vi "Add_Update_Values.vi"(0 "Filename":path, 1 "Value  Constant?":bool, 2 "Edit Raw data files?":bool, 3 "Filetype":string, 5 "New Chs In":string[](array[string])=[""], 7 "Edit Raw Data Header Info":bool, 9 "New Values In":string[][](array[string]), 11 "Selected Rows":i32[](array[numeric]), 12 "Edit all Rows?":bool, 13 "Raw DF in Orig Pos?":bool, 14 "Job Directory":path=path "/G4_2_HD/Users/paulhayden/Documents/Projects/Hong Roughness/XW data/XW_Corr.tpt") -> ()   [LabVIEW 2015]
panel:
  in  "Warn If files not found?":bool=TRUE
  out "Checking Raw data files":i32
  in  "stop":bool
  out "Currently editing":string
  out "Folder Containing Raw data Files":path
  out "size(s)":i32
  out "Files Processed":i32(slide) scale=0.0..522.0
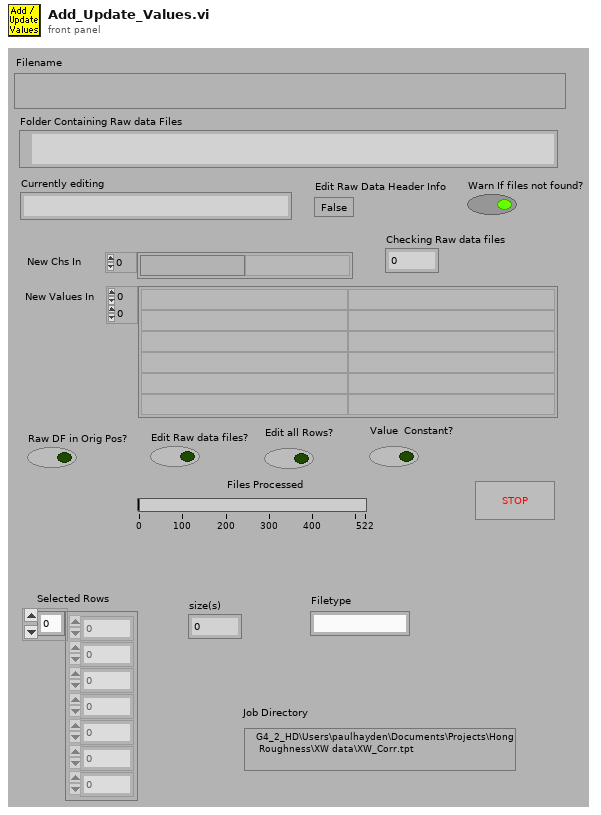
[diagram p1: front panel]
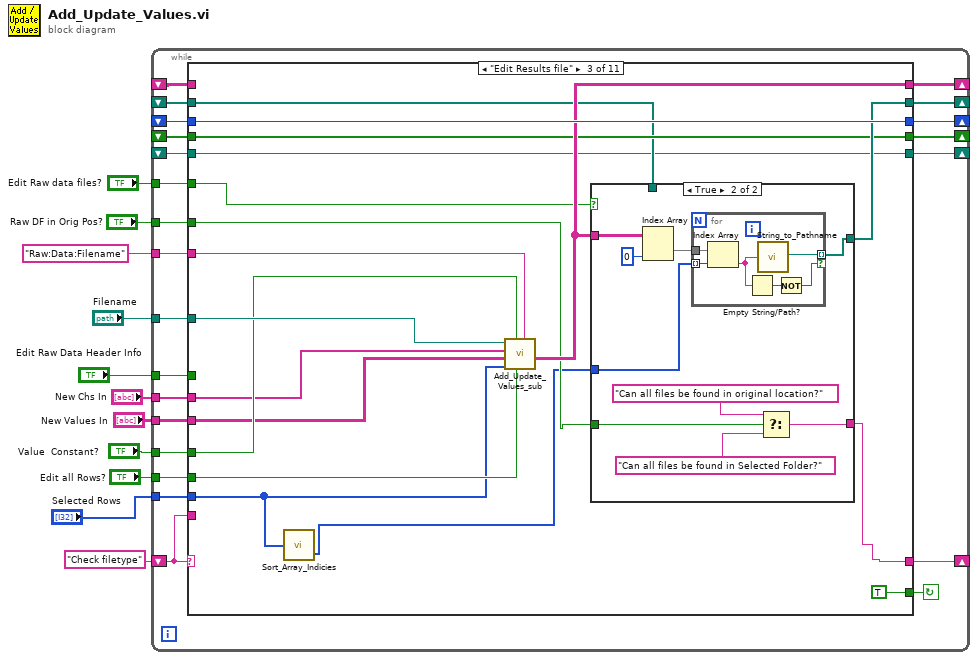
[diagram p0: block diagram]
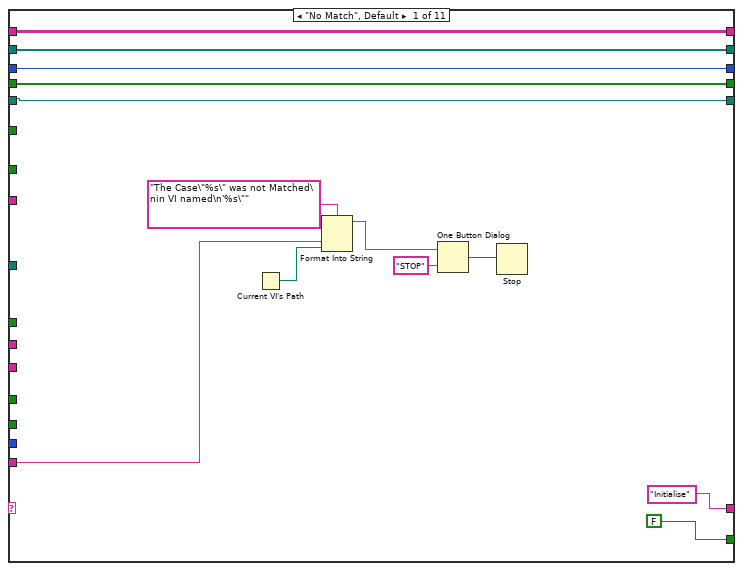
[diagram p2: hidden frame]
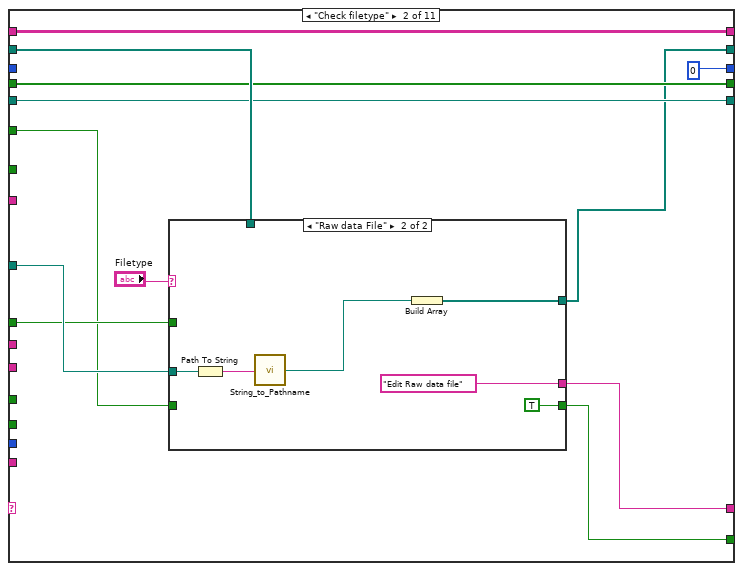
[diagram p3: hidden frame]
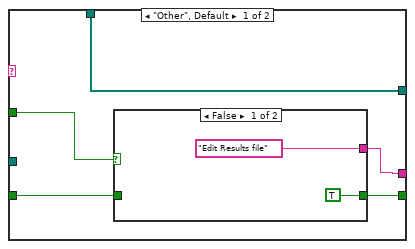
[diagram p4: hidden frame]
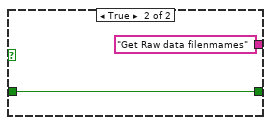
[diagram p5: hidden frame]
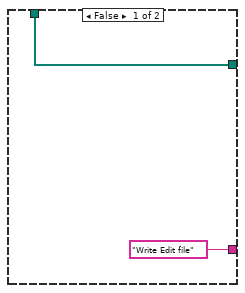
[diagram p6: hidden frame]
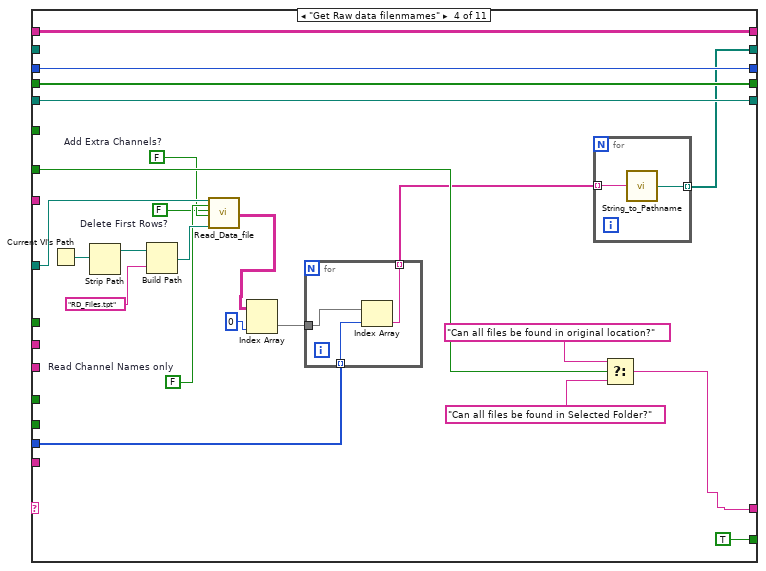
[diagram p7: hidden frame]
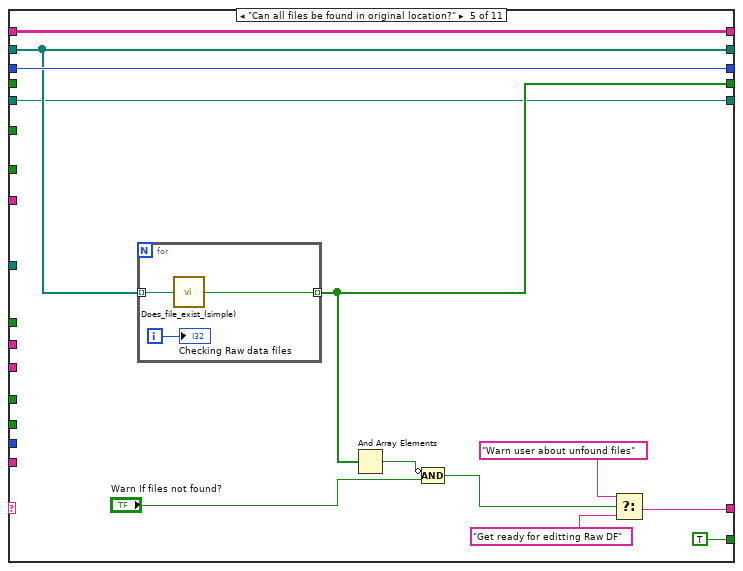
[diagram p8: hidden frame]
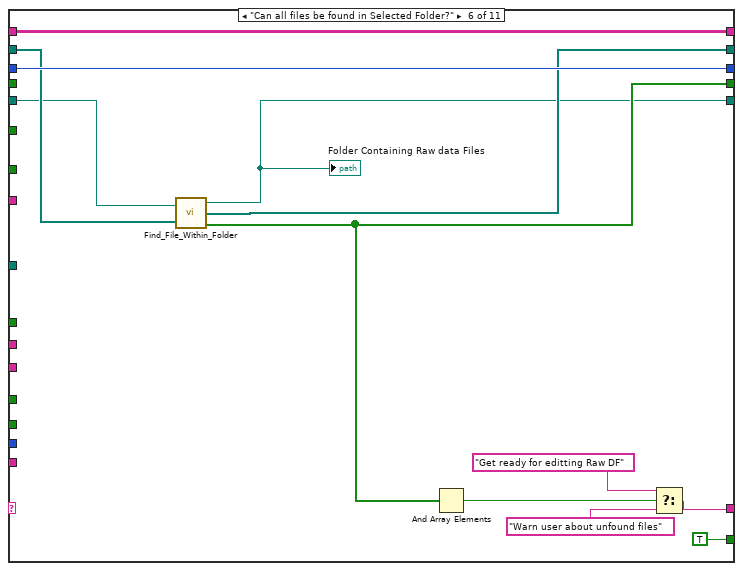
[diagram p9: hidden frame]
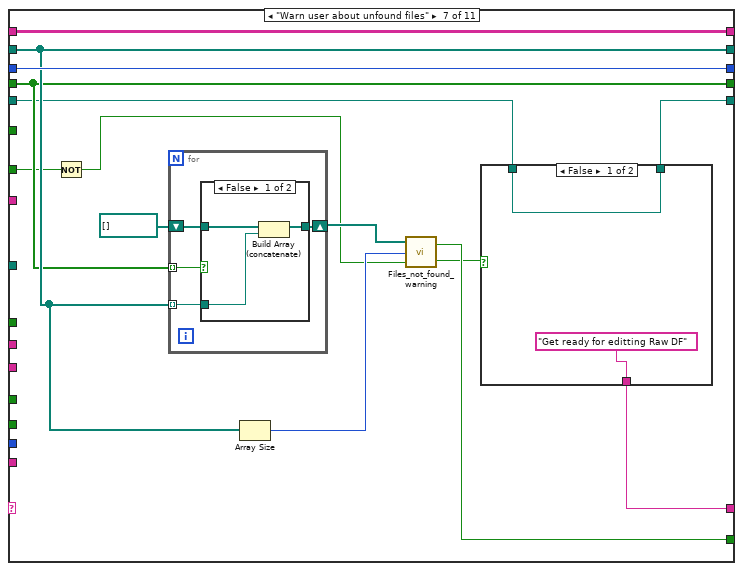
[diagram p10: hidden frame]
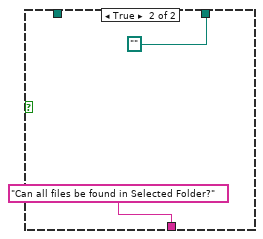
[diagram p11: hidden frame]
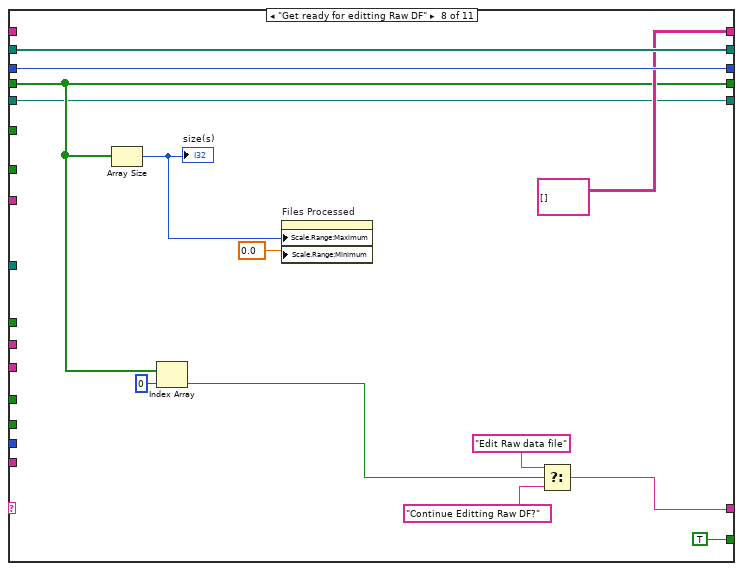
[diagram p13: hidden frame]
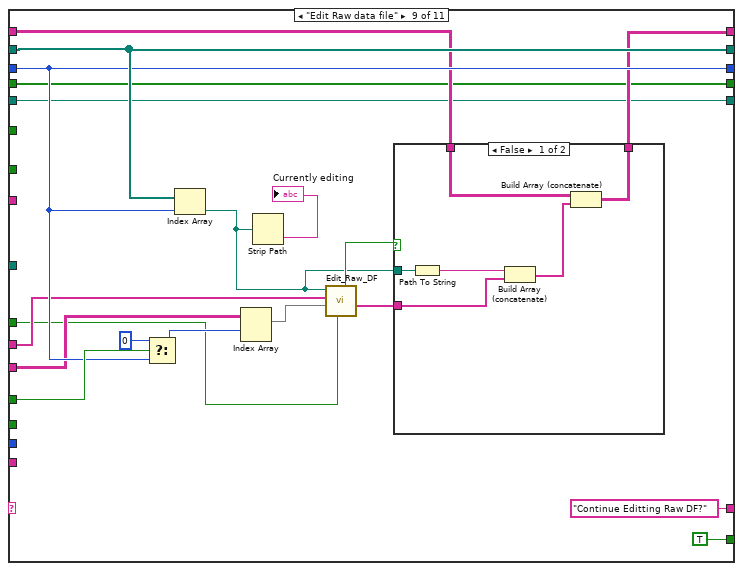
[diagram p14: hidden frame]
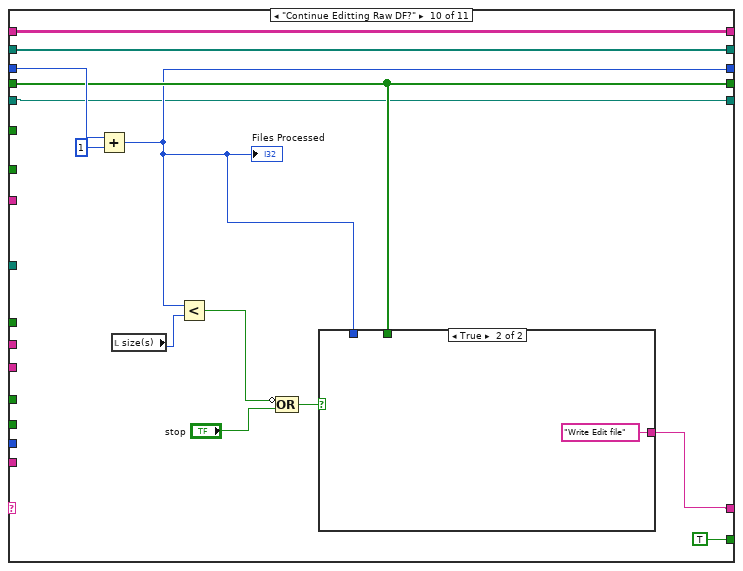
[diagram p16: hidden frame]
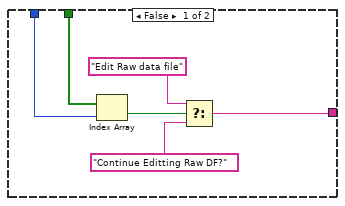
[diagram p17: hidden frame]
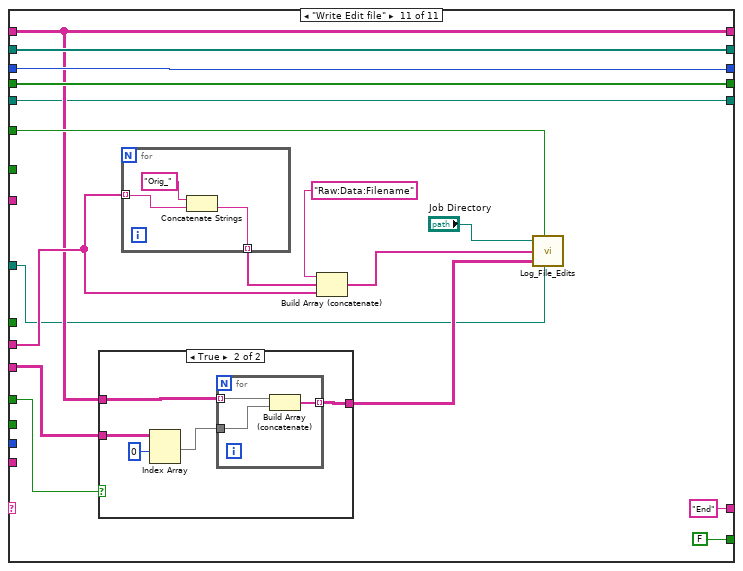
[diagram p18: hidden frame]
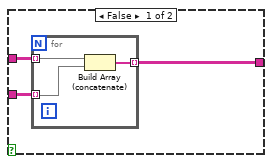
[diagram p19: hidden frame]
diagram:
  n1 = while {
    shift-left: "Check filetype" -> [w32]
    shift-right: [w33] -> _
    shift-right: [w30] -> _
    shift-left: _ -> [w29]
    tunnel: "Filename" -> [w31]
    shift-right: [w28] -> _
    shift-left: _ -> [w27]
    tunnel: "Value  Constant?" -> [w26]
    tunnel: "Edit Raw Data Header Info" -> [w25]
    shift-right: [w24] -> _
    shift-left: _ -> [w23]
    tunnel: "New Chs In" -> [w22]
    tunnel: "New Values In" -> [w21]
    tunnel: "Edit all Rows?" -> [w20]
    shift-right: [w19] -> _
    shift-left: _ -> [w18]
    tunnel: "Edit Raw data files?" -> [w17]
    tunnel: "Raw DF in Orig Pos?" -> [w16]
    shift-right: [w14] -> _
    shift-left: _ -> [w15]
    tunnel: "Selected Rows" -> [w13]
    tunnel: "Raw:Data:Filename" -> [w12]
    stop <- w34 continue-if-true
    n2 = case shown="\"Edit Results file\"" w32 {
      tunnel: [FALSE w50 TRUE TRUE TRUE TRUE w172 TRUE TRUE TRUE FALSE] -> w34
      tunnel: ["Initialise" w57 w81 w129 w144 w155 w168 w195 "Continue Editting Raw DF?" ("t") w234 "End" ("t")] -> w33
      tunnel: w32 -> [w42 _ _ _ _ _ _ _ _ _ _]
      tunnel: w31 -> [_ w55 w90 w118 _ _ _ _ _ _ w252]
      tunnel: [w38 w48 w84 w112 w147 w161 w174 w201 w219 w240 w265] -> w30
      tunnel: w29 -> [w38 w58 w80 _ w147 w160 w174 w201 w219 w240 w265]
      tunnel: [w39 0 w92 w132 w149 w164 w178 w203 w218 w235 w263] -> w28
      tunnel: w27 -> [w39 _ w92 w132 w149 w164 w178 w203 w218 w239 w263]
      tunnel: w26 -> [_ _ w89 _ _ _ _ _ w222 _ w253]
      tunnel: w25 -> [_ w51 _ _ _ _ _ _ w204 _ _]
      tunnel: [w37 w54 w85 w124 w146 w162 w176 string[][] [] ("Edit Info") w209 w241 w256] -> w24
      tunnel: w23 -> [w37 w54 _ w124 w146 w162 w176 _ w210 w241 w256]
      tunnel: w22 -> [_ _ w88 _ _ _ _ _ w216 _ w258]
      tunnel: w21 -> [_ _ w87 _ _ _ _ _ w215 _ w255]
      tunnel: w20 -> [_ _ w86 _ _ _ _ _ _ _ _]
      tunnel: [w36 w53 w83 w130 w145 w156 w173 w199 w208 w236 w264] -> w19
      tunnel: w18 -> [w36 w53 w83 w130 _ _ w173 w199 w208 w236 w264]
      tunnel: w17 -> [_ w49 w82 _ _ _ _ _ _ _ w260]
      tunnel: w16 -> [_ _ w79 w128 _ _ w171 _ _ _ _]
      tunnel: w15 -> [w35 w52 w78 w127 w143 w154 w165 w191 w205 w230 w250]
      tunnel: [w35 w52 w78 w127 w143 w153 w166 w191 w205 w230 w250] -> w14
      tunnel: w13 -> [_ _ w76 w123 _ _ _ _ _ _ _]
      tunnel: w12 -> [_ _ w77 _ _ _ _ _ _ _ _]
      frame "No Match", Default {
        n3 = Current VI's Path() -> (path=w41:path)
        n4 = Format Into String(format string="The Case\"%s\" was not Matched\nin VI named\n'%s\"" ("Format String"), w42, w41) -> (resulting string=w45:string)  [unwired: 2 in, 1 out]
        n5 = One Button Dialog(message=w45, button name ("OK")="STOP") -> (true=w43:bool)
        n6 = Stop(stop? (T)=w43) -> ()
      }
      frame "Check filetype" {
        n7 = case shown="\"Raw data File\"" "Filetype" {
          tunnel: w55 -> [_ w71]
          tunnel: [w64 w74] -> w48
          tunnel: w58 -> [w64 _]
          tunnel: [w62 "Edit Raw data file"] -> w57
          tunnel: w51 -> [w63 _]
          tunnel: [w61 TRUE ("Edit Raw data files?")] -> w50
          tunnel: w49 -> [w60 _]
          frame "Other", Default {
            n8 = case shown="False" w63 {
              tunnel: ["Edit Results file" "Get Raw data filenmames"] -> w62
              tunnel: [TRUE ("Edit Raw data files?") w67] -> w61
              tunnel: w60 -> [_ w67]
              frame False {
              }
              frame True {
              }
            }
          }
          frame "Raw data File" {
            n9 = Path To String(path=w71) -> (string=w70:string)
            n10 = call "String_to_Pathname.vi"("Input String"=w70) -> ("path"=w69:path)
            n11 = Build Array(w69) -> (w74:path[])
          }
        }
      }
      frame "Edit Results file" {
        n12 = call "Sort_Array_Indicies.vi"("unsorted array"=w76) -> ("Sort Index"=w75:i32[])  [unwired: 1 out]
        n13 = call "Add_Update_Values_sub.vi"("Raw data Filename column name"=w77, "Edit all Rows?"=w86, "Value  Constant?"=w89, "Selected Rows"=w76, "New Values In"=w87, "New Chs In"=w88, "Filename"=w90) -> ("Edit Info"=w85:string[][])  [unwired: 4 out]
        n14 = case shown="True" w82 {
          tunnel: w85 -> [_ w103]
          tunnel: [w93 w97] -> w84
          tunnel: w79 -> [_ w101]
          tunnel: ["Write Edit file" w98] -> w81
          tunnel: w80 -> [w93 _]
          tunnel: w75 -> [_ w95]
          frame False {
          }
          frame True {
            n15 = Index Array(array=w103, index (col)=0 ("disabled index (col)")) -> (element=w96:string[])  [unwired: 1 in]
            n16 = for {
              tunnel: [w109] -> w97 mode=indexing if=w104
              tunnel: w96 -> [w108]
              tunnel: w95 -> [w107] mode=indexing
              n17 = Index Array(array=w108, index=w107) -> (element=w106:string)
              n18 = Empty String/Path?(string/path=w106) -> (empty?=w105:bool)
              n19 = call "String_to_Pathname.vi"("Input String"=w106) -> ("path"=w109:path)
              n20 = Not(x=w105) -> (.not. x?=w104:bool)
            }
            n21 = Select(t="Can all files be found in original location?", s=w101, f="Can all files be found in Selected Folder?") -> (s? t:f=w98:string)
          }
        }
      }
      frame "Get Raw data filenmames" {
        w110 = FALSE  # Delete First Rows?
        w115 = FALSE  # Add Extra Channels?
        w116 = FALSE  # Read Channel Names only
        n22 = Current VI's Path() -> (path=w121:path)
        n23 = Strip Path(path=w121) -> (stripped path=w120:path)  [unwired: 1 out]
        n24 = Build Path(base path=w120, name or relative path="RD_Files.tpt") -> (appended path=w117:path)
        n25 = call "Read_Data_file.vi"("Results file"=w118, "Read Channel Names only"=w116, "Delete First Rows?"=w110, "Add Extra Channels?"=w115, "Template File"=w117) -> ("Channel Values Out"=w114:string[][])  [unwired: 1 in, 13 out]
        n26 = Index Array(array=w114, index (col)=0 ("index (row)")) -> (element=w122:string[])  [unwired: 1 in]
        n27 = for {
          tunnel: w123 -> [w137] mode=indexing
          tunnel: w122 -> [w136]
          tunnel: [w135] -> w111 mode=indexing
          n28 = Index Array(array=w136, index=w137) -> (element=w135:string)
        }
        n29 = for {
          tunnel: [w134] -> w112 mode=indexing
          tunnel: w111 -> [w133] mode=indexing
          n30 = call "String_to_Pathname.vi"("Input String"=w133) -> ("path"=w134:path)
        }
        n31 = Select(t="Can all files be found in original location?", s=w128, f="Can all files be found in Selected Folder?") -> (s? t:f=w129:string)
      }
      frame "Can all files be found in original location?" {
        n32 = for {
          tunnel: w147 -> [w152] mode=indexing
          tunnel: [w151] -> w145 mode=indexing
          i -> [w150]
          n33 = call "Does_file_exist_(simple).vi"("Pathname"=w152) -> ("exists?"=w151:bool)
          "Checking Raw data files" <- w150
        }
        n34 = And Array Elements(Boolean array=w145) -> (logical AND=w142:bool)
        n35 = Compound Arithmetic op=AND(invert w142, "Warn If files not found?") -> (w140:bool)
        n36 = Select(t="Warn user about unfound files", s=w140, f="Get ready for editting Raw DF" ("t")) -> (s? t:f=w144:string)
      }
      frame "Can all files be found in Selected Folder?" {
        n37 = call "Find_File_Within_Folder.vi"("Folder to Search"=w154, "Files to find"=w160) -> ("Folder to Search Out"=w153:path, "New File Paths"=w161:path[], "Files Found?"=w156:bool[])
        "Folder Containing Raw data Files" <- w153
        n38 = And Array Elements(Boolean array=w156) -> (logical AND=w159:bool)
        n39 = Select(t="Get ready for editting Raw DF", s=w159, f="Warn user about unfound files") -> (s? t:f=w155:string)
      }
      frame "Warn user about unfound files" {
        n40 = Not(x=w171) -> (.not. x?=w170:bool)
        n41 = for {
          tunnel: w174 -> [w183] mode=indexing
          shift-right: [w186] -> w175
          shift-left: path[] [] -> [w185]
          tunnel: w173 -> [w184] mode=indexing
          n42 = case shown="False" w184 {
            tunnel: w185 -> [w189 w190]
            tunnel: [w187 w190] -> w186
            tunnel: w183 -> [w188 _]
            frame False {
              n43 = Build Array (concatenate)(w189, w188) -> (w187:path[])
            }
            frame True {
            }
          }
        }
        n44 = Array Size(array=w174) -> (size(s)=w177:i32)
        n45 = call "Files_not_found_warning.vi"("Use Selected Folder?"=w170, "Total number of data files"=w177, "Unfound Files"=w175) -> ("Edit Selected Folder Out"=w169:bool, "Edit Files?"=w172:bool)
        n46 = case shown="False" w169 {
          tunnel: ["Get ready for editting Raw DF" ("t") "Can all files be found in Selected Folder?" ("t")] -> w168
          tunnel: [w179 path ""] -> w166
          tunnel: w165 -> [w179 _]
          frame False {
          }
          frame True {
          }
        }
      }
      frame "Get ready for editting Raw DF" {
        n47 = Array Size(array=w199) -> (size(s)=w192:i32)
        "size(s)" <- w192
        n48 = Index Array(array=w199, index=0) -> (element=w197:bool)
        n49 = property on="Files Processed" class="Slide (strict)"("Scale.Range:Maximum"=w192, "Scale.Range:Minimum"=0.0 ("Scale.Range:Maximum")) -> ()  [unwired: 2 in, 2 out]
        n50 = Select(t="Edit Raw data file", s=w197, f="Continue Editting Raw DF?") -> (s? t:f=w195:string)
      }
      frame "Edit Raw data file" {
        n51 = Select(t=0, s=w222, f=w218) -> (s? t:f=w220:i32)
        n52 = Index Array(array=w219, index=w218) -> (element=w207:path)
        n53 = Index Array(array=w215, index (row)=w220) -> (element=w214:string[])  [unwired: 1 in]
        n54 = Strip Path(path=w207) -> (name=→"Currently editing":string)  [unwired: 1 out]
        n55 = call "Edit_Raw_DF.vi"("Edit Raw Data Header Info"=w204, "New Values In"=w214, "New Chs In"=w216, "Data filename"=w207) -> ("Original values"=w212:string[], "File Not Changed?"=w211:bool)  [unwired: 2 in, 2 out]
        n56 = case shown="False" w211 {
          tunnel: w207 -> [w228 _]
          tunnel: w212 -> [w226 _]
          tunnel: w210 -> [w224 w229]
          tunnel: [w223 w229] -> w209
          frame False {
            n57 = Path To String(path=w228) -> (string=w227:string)
            n58 = Build Array (concatenate)(w227, w226) -> (w225:string[])
            n59 = Build Array (concatenate)(w224, w225) -> (w223:string[][])
          }
          frame True {
          }
        }
      }
      frame "Continue Editting Raw DF?" {
        n60 = Add(x=w239, y=1) -> (x+y=w235:i32)
        "Files Processed" <- w235
        n61 = local read "size(s)"() -> (w237:i32)
        n62 = Less?(x=w235, y=w237) -> (x < y?=w232:bool)
        n63 = Compound Arithmetic op=OR(invert w232, "stop") -> (w231:bool)
        n64 = case shown="True" w231 {
          tunnel: w236 -> [w247 _]
          tunnel: w235 -> [w246 _]
          tunnel: [w244 "Write Edit file" ("t")] -> w234
          frame False {
            n65 = Index Array(array=w247, index=w246) -> (element=w248:bool)
            n66 = Select(t="Edit Raw data file", s=w248, f="Continue Editting Raw DF?") -> (s? t:f=w244:string)
          }
          frame True {
          }
        }
      }
      frame "Write Edit file" {
        n67 = case shown="True" w253 {
          tunnel: w256 -> [w269 w277]
          tunnel: w255 -> [w268 w275]
          tunnel: [w267 w276] -> w254
          frame False {
            n68 = for {
              tunnel: w269 -> [w272] mode=indexing
              tunnel: w268 -> [w271] mode=indexing
              tunnel: [w270] -> w267 mode=indexing
              n69 = Build Array (concatenate)(w272, w271) -> (w270:string[])
            }
          }
          frame True {
            n70 = Index Array(array=w275, index (row)=0) -> (element=w273:string[])  [unwired: 1 in]
            n71 = for {
              tunnel: w277 -> [w280] mode=indexing
              tunnel: [w279] -> w276 mode=indexing
              tunnel: w273 -> [w278]
              n72 = Build Array (concatenate)(w280, w278) -> (w279:string[])
            }
          }
        }
        n73 = for {
          tunnel: w258 -> [w283] mode=indexing
          tunnel: [w281] -> w259 mode=indexing
          n74 = Concatenate Strings("Orig_" ("string"), w283) -> (w281:string)
        }
        n75 = Build Array (concatenate)("Raw:Data:Filename", w259, w258) -> (w257:string[])
        n76 = call "Log_File_Edits.vi"("Job Directory"="Job Directory", "File Editted?"=w260, "Channels to Edit"=w257, "Data"=w254, "Results file name"=w252) -> ()  [unwired: 2 out]
      }
    }
  }
